vi "calculate_Ud_estimate.vi"(0 "Tau_ch":dbl[](array[numeric])=[0.11491729291343579, 0.11716798919571741, 0.11740631364396965, 0.11663726342199245, 0.41599980468961384, 0.11981011551839264, 0.11846429840933606, 0.11867732465684001, 0.1099546558688366, 0.11157519276959196, 0.10652596659944064, 0.11187533014192738, 0.11242534122168901, 0.11250590452650158, 0.11233958629056463, 0.11088956837703348, 0.11684290859752998, 0.11711408209103276, 0.11862962903855054, 0.11574688850921441, 0.11080958640139682, 0.11308007616237671, 0.11316833203019577, 0.11732662567656041, 0.11776955995449861, 0.11488434870753593, 0.11721346913661516, 0.11723600482803162, 0.1173219143188469, 0.11486538187917118, 0.1161354905419326, 0.11580597702447244, 0.11089805083278159, 0.10965173450878267, 0.10989266890532523, 0.11049724960692761, 0.11094253276914103, 0.1112015939579455, 0.11056511595580205, 0.11125203268352817, 0.10851766683731974, 0.10665739286095859, 0.10665088457538054, 0.10647759616581123, 0.10805487600009084, 0.10533289893772232, 0.10446227511758968, 0.10416638033440741, 0.11156846805821136, 0.11129308727212155, 0.11117840263008584, 0.1102971572868625, 0.10837301568677209, 0.11586325578254852, 0.11338638335503164, 0.11266837385466463, 0.11020464539493718, 0.11718312222258088, 0.11005940383900907, 0.11074035298635442, 0.11310264754168789, 0.11428021968521139, 0.10890693978140649, 0.11304857784773828, 0.11071164775178235, 0.10899043148625223, 0.1098152132889097, 0.11071094104034687, 0.10922727710545306, 0.11026461123495493, 0.10902110264823185, 0.1063818330991493, 0.1082901421909468, 0.10855104773097228, 0.10976304069098969, 0.1092806529611063, 0.10813898027014157, 0.10856892511543396, 0.10528805150138838, 0.10996755406311447, 0.11441717863822966, 0.11512938300201939, 0.11354812708860414, 0.11170183444428032, 0.10929951535815542, 0.10880924561891742, 0.11032002393110663, 0.12233406623444484, 0.10819046523889579, 0.10676534101945172, 0.11334069041654328, 0.11395839570756812, 0.10860855876008385, 0.11000092792604536, 0.11150855742531308, 0.11072296835591808, 0.11248944715419666, 0.11109385151927784, 0.10904702395407219, 0.0, 0.11012618939531567, 0.1101228599630128, 0.10901646637252452, 0.10848342666256441, 0.1118672405375629, 0.11165093132257785, 0.11030651312297526, 0.1105637825970819, 0.10972695234743621, 0.11008183794997571, 0.10869604711918752, 0.0, 0.10947241009391531, 0.5898071300815099, 0.41732939048318163, 0.0, 0.0, 0.0, 0.0, 0.0, 0.0, 0.0, 0.5051635137410128, 0.0, 0.0, 0.0, 0.4056247218989413, 0.0, 0.11491729291343579], 1 "kbolott_and_volume":dbl[][](array[numeric]), 2 "Kappa_ch":dbl[](array[numeric])=[0.0008402794220111138, 0.0008162628511746609, 0.0008306690902202418, 0.000803901120831155, 0.0003482758920990883, 0.0008106589659042871, 0.0008016286027972057, 0.000799559666964026, 0.0008329596140242245, 0.0008550459829924856, 0.0007662506038997399, 0.0008054791716010769, 0.0008538518247154832, 0.0008293547031323884, 0.0008561853513376051, 0.0008533408283799155, 0.0008374094293251158, 0.0008246891754373999, 0.0008094405414334474, 0.0008290847564626268, 0.00020601047667132065, 0.000800173048893566, 0.0007793179002779764, 0.0007971071724399289, 0.0007885266906587188, 0.0007777314742190596, 0.000805938950941268, 0.0007876903707101731, 0.0008486502743123638, 0.0008188176160358826, 0.0008275575494250777, 0.0008021526930523769, 0.0004219866202355569, 0.0008028836567896177, 0.0007965332650444257, 0.0007657694302588966, 0.0007891955147847732, 0.0007918255330716038, 0.0007896451983246505, 0.0007639621417921391, 0.0008241807402430576, 0.0008494655305824806, 0.0008513286284044697, 0.0008584599469876866, 0.0008065529851855167, 0.0008583681445476364, 0.0008848769105909991, 0.0008824761623272339, 0.0008739299904558458, 0.0008726933272884011, 0.0008591817798513973, 0.0008546408142867519, 0.0008814192063552359, 0.000837962132357275, 0.0008754373245495078, 0.0008659455513111399, 0.000875854800823488, 0.0008145627712648352, 0.000847096348180231, 0.0008354027185001123, 0.0008988684127044384, 0.0009087972104601418, 0.000872460372055295, 0.0008865774530667089, 0.0008205858447961992, 0.0008661153610700915, 0.0008514123741077071, 0.0008674455175914637, 0.0008535020874821334, 0.0008530135268333135, 0.0008817680910658127, 0.0008857682842425993, 0.0009014333315122717, 0.0009058705470039874, 0.0009451074888355545, 0.0008658347728111954, 0.0008865415114476586, 0.0009037142514292518, 0.0009300212486309693, 0.0009201252229947723, 0.0008662494433570838, 0.0008561155107896092, 0.0008934103962644251, 0.000843038472812381, 0.0008821165464311927, 0.0008725326170488139, 0.0008607956284658778, 0.0008692253024054895, 0.0007600922149492939, 0.0007595503979645458, 0.0008808740943017723, 0.0008427393057336779, 0.0008151549367042052, 0.0008178123459529788, 0.0008143006723436752, 0.0008042217964108747, 0.0007735257506859799, 0.0007705827889143488, 0.0007855750338204015, 1.5378016423296697e-10, 0.0007777843483157151, 0.0007914940873736198, 0.0007883969825026242, 0.000818379256343944, 0.0008183032224836934, 0.0008253700992517207, 0.0008193590844345892, 0.0008108478163956726, 0.0007992276276126246, 0.0007886605041422787, 0.000781928010070813, 1.3117348375603198e-11, 0.0007692233287415738, -6.433477601629483e-12, 5.840652071940865e-11, -5.095362431956802e-12, 1.483332911600832e-10, -2.3650890104320048e-11, 2.0638470359814695e-11, -4.2942497083098924e-12, -1.609109206826474e-13, -8.281241741308274e-13, -1.484842606490482e-11, 1.312154360785075e-10, -1.3280672580076002e-10, 3.875382814091509e-11, -5.840342459280051e-12, 1.6602972107316198e-05], 3 "F_ch":dbl[](array[numeric]), 4 "SampleTime":sgl=0.0008, 5 "tau_fact":dbl[](array[numeric]), 6 "estimated floating voltage":dbl format="%#_13g", 7 "Offset (V)":dbl[](array[numeric]), 8 "elected channel for output":i32) -> (16 "voltage factor":dbl, 17 "estimated voltage":dbl)   [LabVIEW 2014]
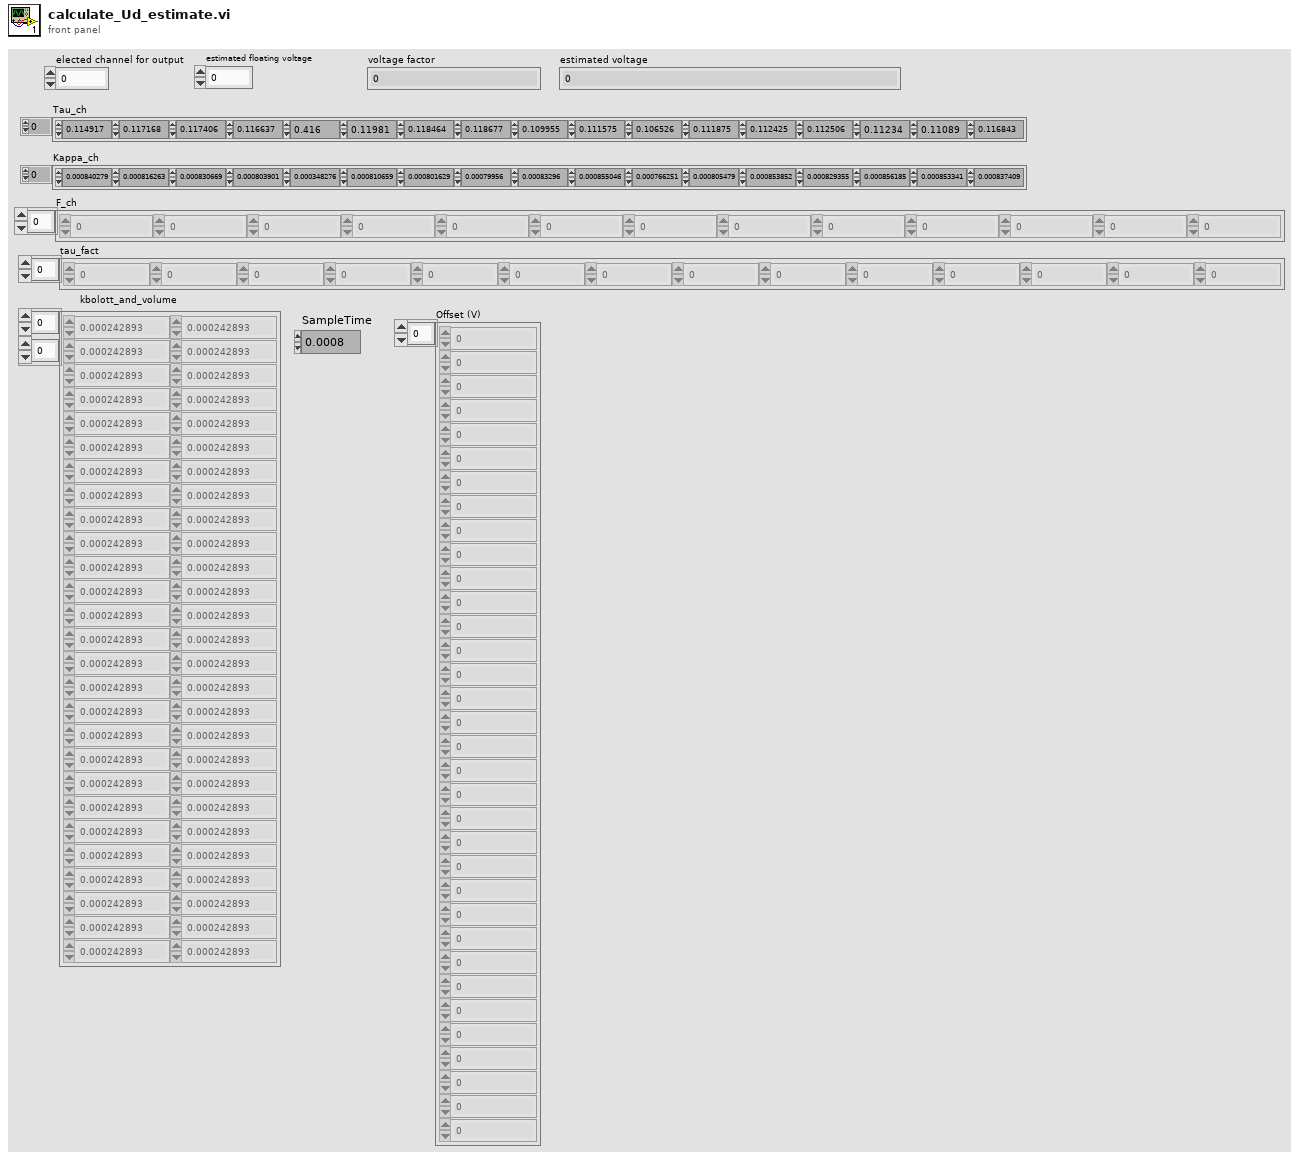
[diagram p1: front panel]
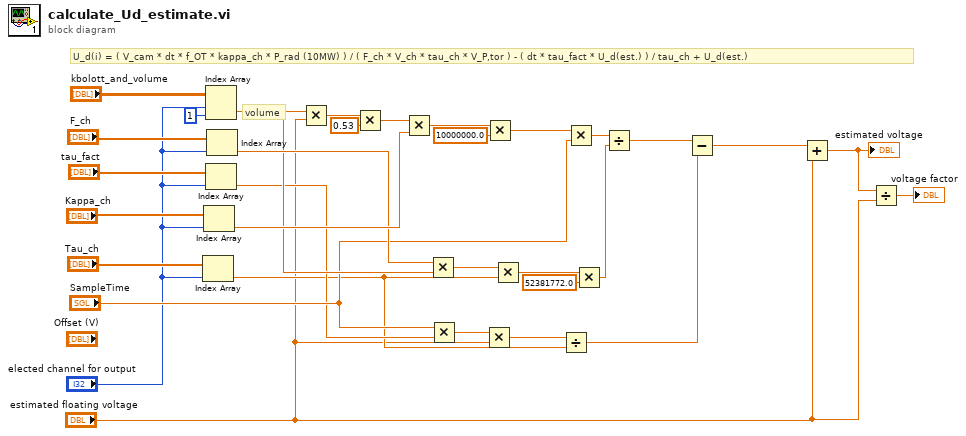
[diagram p0: block diagram]
diagram:
  # "volume"
  # "U_d(i) = ( V_cam * dt * f_OT * kappa_ch * P_rad (10MW) ) / ( F_ch * V_ch * tau_ch * V_P,tor ) - ( dt * tau_fact * U_d(est.) ) / tau_ch + U_d(est.)"
  n1 = Index Array(array="Tau_ch", index="elected channel for output") -> (element=w6:dbl)
  n2 = Index Array(array="Kappa_ch", index="elected channel for output") -> (element=w26:dbl)
  n3 = Index Array(array="kbolott_and_volume", index (row)="elected channel for output", index (col)=1 ("disabled index (col)")) -> (element=w21:dbl)
  n4 = Index Array(array="tau_fact", index="elected channel for output") -> (element=w9:dbl)
  n5 = Index Array(array="F_ch", index="elected channel for output") -> (element=w22:dbl)
  n6 = Multiply(x=w21, y="estimated floating voltage") -> (x*y=w30:dbl)
  n7 = Multiply(x=w30, y=0.53) -> (x*y=w28:dbl)
  n8 = Multiply(x=w28, y=w26) -> (x*y=w25:dbl)
  n9 = Multiply(x=w22, y=w21) -> (x*y=w19:dbl)
  n10 = Multiply(x="SampleTime", y=w9) -> (x*y=w8:dbl)
  n11 = Multiply(x=w8, y="estimated floating voltage") -> (x*y=w7:dbl)
  n12 = Multiply(x=w25, y=10000000.0) -> (x*y=w13:dbl)
  n13 = Multiply(x=w19, y=w6) -> (x*y=w18:dbl)
  n14 = Divide(x=w7, y=w6) -> (x/y=w5:dbl)
  n15 = Multiply(x=w13, y="SampleTime") -> (x*y=w14:dbl)
  n16 = Multiply(x=w18, y=52381772.0) -> (x*y=w16:dbl)
  n17 = Divide(x=w14, y=w16) -> (x/y=w15:dbl)
  n18 = Subtract(x=w15, y=w5) -> (x-y=w4:dbl)
  n19 = Add(x=w4, y="estimated floating voltage") -> (x+y=w3:dbl)
  "estimated voltage" <- w3
  n20 = Divide(x=w3, y="estimated floating voltage") -> (x/y=→"voltage factor":dbl)
